vi "LVIS_VerifyMeas.vi"(8 "Error In":errorcluster, 11 "MeasInfoIn":T1) -> (0 "Error Out":errorcluster, 3 "MeasInfoOut":T1)   [LabVIEW 2015]
doc: "Determines the Measurement Info based on the LVIS_Settings file and passed in values, giving precedence to the file and deriving values where requested."
uses:
  Globals/LVIS_IsGlobal.vi
panel:
  out "DateTime":string
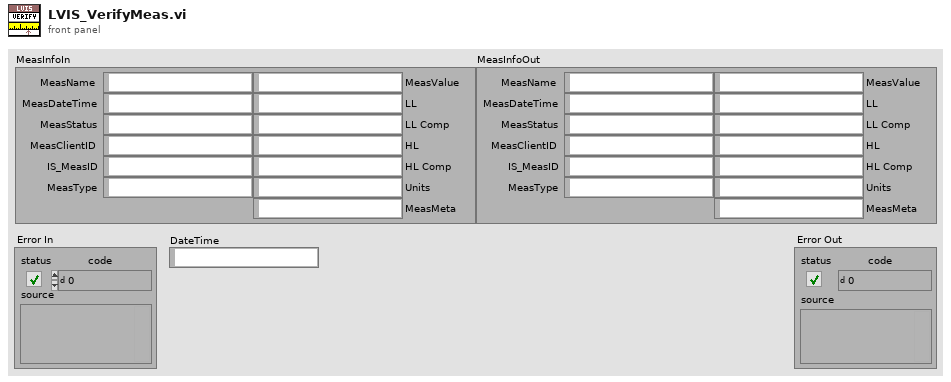
[diagram p1: front panel]
types:
  T1 = cluster{"MeasName":string, "MeasDateTime":string, "MeasStatus":string, "MeasClientID":string, "IS_MeasID":string, "MeasType":string, "MeasValue":string, "LL":string, "LL Comp":string, "HL":string, "HL Comp":string, "Units":string, "MeasMeta":string}
  T2 = cluster{"[0]":string, "[1]":string, "[2]":string, "[3]":string, "[4]":string, "[5]":string, "[6]":string, "[7]":string, "[8]":string, "[9]":string, "[10]":string, "[11]":string, "[12]":string}
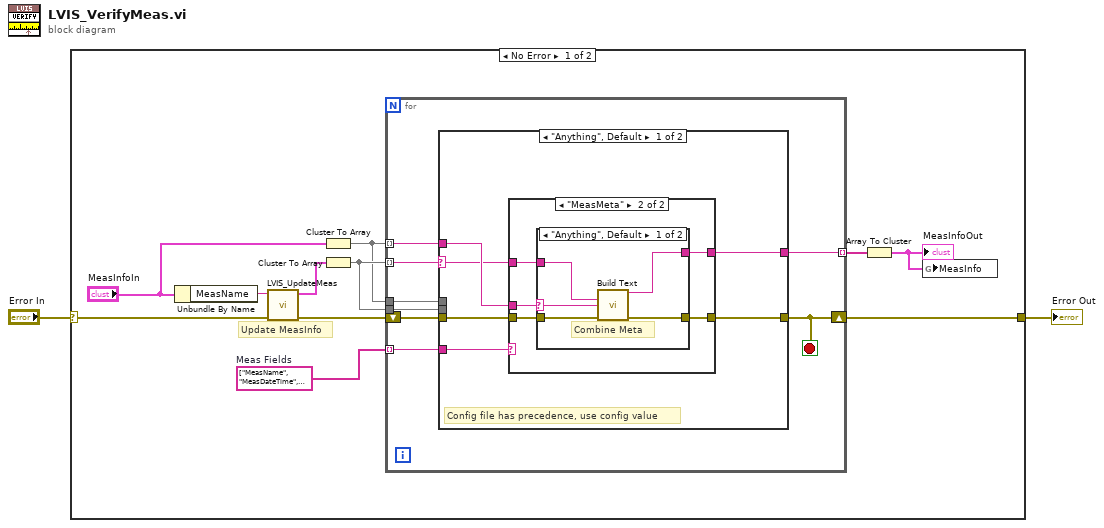
[diagram p0: block diagram]
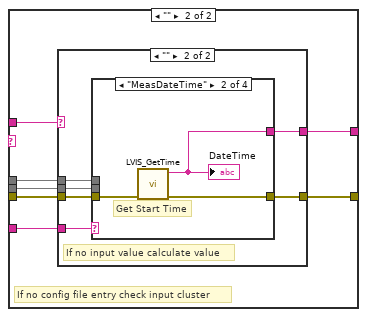
[diagram p4: hidden frame]
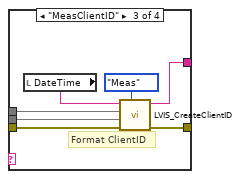
[diagram p7: hidden frame]
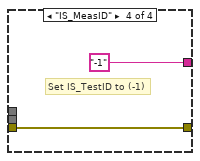
[diagram p8: hidden frame]
diagram:
  n1 = case shown="No Error" "Error In" {
    selector: "Error In" -> [w13 w70]
    tunnel: [w12 w70] -> w1
    frame No Error {
      w3 = string[] ["MeasName", "MeasDateTime", "MeasStatus", "MeasClientID", "IS_MeasID", "MeasType", "MeasValue", "LL", "LL Comp", "HL", "HL Comp", "Units", "MeasMeta"]  # Meas Fields
      # "Update MeasInfo"
      n2 = Unbundle By Name("MeasInfoIn") -> ("MeasName"=w8:string)
      n3 = call "LVIS_UpdateMeas.vi"("Error In"=w13, "MeasName"=w8) -> ("Error out"=w10:errorcluster, "MeasInfo"=w9:T1)  [unwired: 8 in]
      n4 = Cluster To Array(cluster="MeasInfoIn") -> (array=w6:string[])
      n5 = Cluster To Array(cluster=w9) -> (array=w7:string[])
      n6 = for {
        tunnel: w7 -> [w20] mode=indexing
        tunnel: w3 -> [w18] mode=indexing
        shift-right: [w17] -> w12
        shift-left: w10 -> [w21]
        tunnel: w6 -> [w19] mode=indexing
        tunnel: [w16] -> w11 mode=indexing
        tunnel: w7 -> [w15]
        tunnel: w6 -> [w14]
        stop <- w17 stop-if-true
        n7 = case shown="\"Anything\", Default" w20 {
          selector: w20 -> [w22 _]
          tunnel: w21 -> [w26 w47]
          tunnel: [w25 w46] -> w17
          tunnel: [w23 w45] -> w16
          tunnel: w18 -> [w27 w44]
          tunnel: w19 -> [w24 w48]
          tunnel: w15 -> [_ w43]
          tunnel: w14 -> [_ w42]
          frame "Anything", Default {
            # "Config file has precedence, use config value"
            n8 = case shown="\"MeasMeta\"" w27 {
              tunnel: w26 -> [w29 w34]
              tunnel: [w29 w33] -> w25
              tunnel: w24 -> [_ w31]
              tunnel: [w28 w32] -> w23
              tunnel: w22 -> [w28 w30]
              frame "Other", Default {
                # "Non-Meta Config Data"
              }
              frame "MeasMeta" {
                n9 = case shown="\"Anything\", Default" w31 {
                  selector: w31 -> [w35 _]
                  tunnel: w34 -> [w39 w40]
                  tunnel: [w38 w40] -> w33
                  tunnel: [w37 w41] -> w32
                  tunnel: w30 -> [w36 w41]
                  frame "Anything", Default {
                    # "Combine Meta"
                    n10 = call "Build Text"("Meta1"=w36, "Meta2"=w35, "error in (no error)"=w39) -> ("Result"=w37:string, "error out"=w38:errorcluster)  [unwired: 11 in]
                  }
                  frame "" {
                    # "No passed in Meta"
                  }
                }
              }
            }
          }
          frame "" {
            # "If no config file entry check input cluster"
            n11 = case shown="\"\"" w48 {
              selector: w48 -> [w49 _]
              tunnel: w47 -> [w50 w56]
              tunnel: [w50 w54] -> w46
              tunnel: [w49 w53] -> w45
              tunnel: w44 -> [_ w55]
              tunnel: w43 -> [_ w52]
              tunnel: w42 -> [_ w51]
              frame "Anything", Default {
                # "Use input cluster value"
              }
              frame "" {
                # "If no input value calculate value"
                n12 = case shown="\"MeasDateTime\"" w55 {
                  tunnel: w56 -> [w57 w60 w67 w68]
                  tunnel: [w57 w59 w66 w68] -> w54
                  tunnel: [_ w58 w64 "-1" ("ClientID")] -> w53
                  tunnel: w52 -> [_ _ w62 _]
                  tunnel: w51 -> [_ _ w61 _]
                  frame "Other", Default {
                    # "Value is not calculated"
                  }
                  frame "MeasDateTime" {
                    # "Get Start Time"
                    n13 = call "LVIS_GetTime.vi"("Error In"=w60) -> ("Error out"=w59:errorcluster, "DateTime"=w58:string)  [unwired: 9 in]
                    "DateTime" <- w58
                  }
                  frame "MeasClientID" {
                    # "Format ClientID"
                    n14 = local read "DateTime"() -> (w65:string)
                    n15 = call "LVIS_CreateClientID.vi"("Type"=enum16{"Event", "Test", "Meas"}."Meas", "Error In"=w67, "CfgInfo"=w62, "InputInfo"=w61, "DateTime"=w65) -> ("Error out"=w66:errorcluster, "ClientID"=w64:string)  [unwired: 5 in]
                  }
                  frame "IS_MeasID" {
                    # "Set IS_TestID to (-1)"
                  }
                }
              }
            }
          }
        }
      }
      n16 = Array To Cluster(array=w11) -> (cluster=w4:T2)
      "MeasInfoOut" <- w4
      n17 = global write "LVIS_IsGlobal.vi" "MeasInfo"(w4) -> ()
    }
    frame Error {
    }
  }
  "Error Out" <- w1
